vi "TailCut.vi"(8 "error in (no error)":errorcluster, 11 "Snake in":refnum<class "Snake.lvclass">) -> (0 "error out":errorcluster, 3 "Snake out":refnum<class "Snake.lvclass">)   [LabVIEW 2014, in "Snake.lvclass"]
uses:
  Snake.lvclass
  Snake.lvclass/Snake.ctl
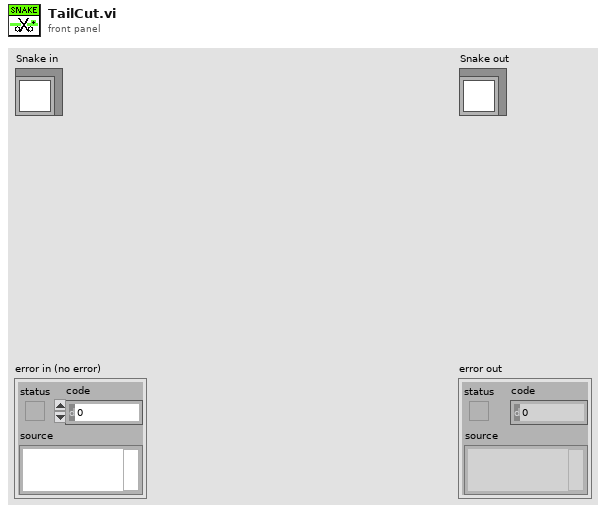
[diagram p1: front panel]
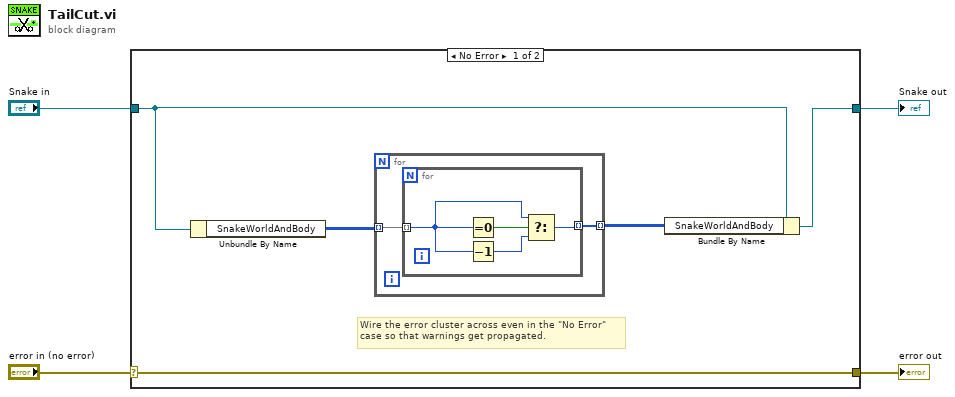
[diagram p0: block diagram]
diagram:
  n1 = case shown="No Error" "error in (no error)" {
    selector: "error in (no error)" -> [w9 w17]
    tunnel: [w9 w17] -> w3
    tunnel: [w8 w16] -> w1
    tunnel: "Snake in" -> [w7 w16]
    frame No Error {
      # "Wire the error cluster across even in the \"No Error\"\ncase so that warnings get propagated."
      n2 = Unbundle By Name(w7) -> ("SnakeWorldAndBody"=w6:u32[][])
      n3 = for {
        tunnel: w6 -> [w11] mode=indexing
        tunnel: [w10] -> w5 mode=indexing
        n4 = for {
          tunnel: w11 -> [w12] mode=indexing
          tunnel: [w14] -> w10 mode=indexing
          n5 = Equal To 0?(x=w12) -> (x = 0?=w15:bool)
          n6 = Decrement(x=w12) -> (x-1=w13:u32)
          n7 = Select(t=w12, s=w15, f=w13) -> (s? t:f=w14:u32)
        }
      }
      n8 = Bundle By Name(cluster=w7, "SnakeWorldAndBody"=w5) -> (w8:refnum<class "Snake.lvclass">)
    }
    frame Error {
    }
  }
  "error out" <- w3
  "Snake out" <- w1
